vi "_PC_Daemon_Config_SaveData.vi"(8 "error in (no error)":errorcluster) -> (0 "error out":errorcluster)   [LabVIEW 2018]
uses:
  <vilib>/event_ctls.llb/eventvkey.ctl
panel:
  in  "Apply":bool
  in  "S/N":dbl
  in  "Noise Height":dbl
  in  "Auto Save":bool
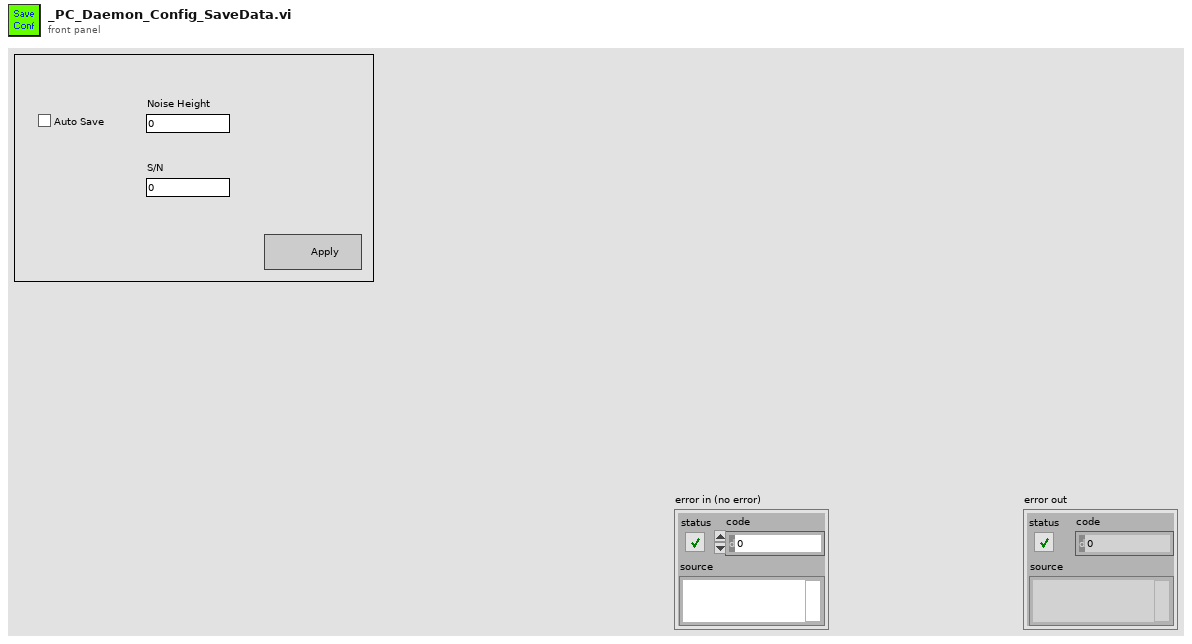
[diagram p1: front panel]
types:
  T1 = enum8{"Enabled", "Disabled", "Disabled and Grayed Out"}
  T2 = typedef "eventvkey.ctl" = enum16{"ASCII", "Enter", "Return", "Shift", "Ctrl", "Alt", "Cmd", "Opt", "Caps", "NumLock", "Clear", "Break", "Up", "Down", "Left", "Right", "Insert", "Delete", "Home", "End", "PageUp", "PageDown", "Escape", "Help", "Pause", "ScrollLock", "F1", "F2", "F3", "F4", "F5", "F6", "F7", "F8", "F9", "F10", "F11", "F12", "F13", "F14", "F15", "F16", "F17", "F18", "F19", "F20", "F21", "F22", "F23", "F24", "Play", "VolumeUp", "VolumeDown", "Mute", "Two Byte Char"}
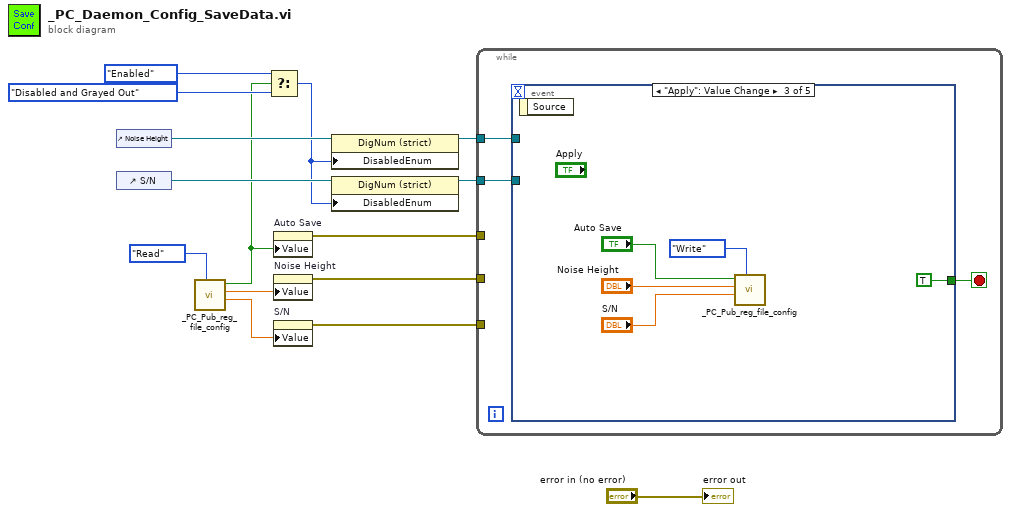
[diagram p0: block diagram]
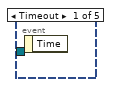
[diagram p2: hidden frame]
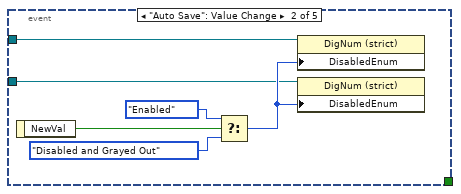
[diagram p3: hidden frame]
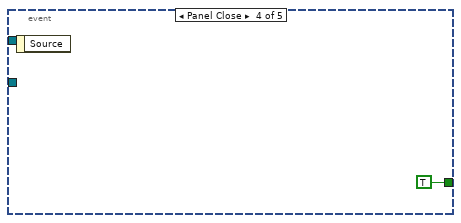
[diagram p4: hidden frame]
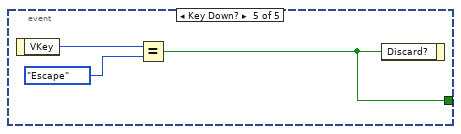
[diagram p5: hidden frame]
diagram:
  n1 = control-ref of="Noise Height"() -> (w8:refnum<vi>)
  n2 = control-ref of="S/N"() -> (w7:refnum<vi>)
  n3 = call "_PC_Pub_reg_file_config.vi"("func"=enum16{"None", "Write", "Read"}."Read") -> ("FileSN out"=w9:sgl, "FileNoise out"=w10:dbl, "AutoSave out"=w2:bool)  [unwired: 4 in, 1 out]
  n4 = Select(t=T1."Enabled" ("Disabled"), s=w2, f=T1."Disabled and Grayed Out" ("Disabled")) -> (s? t:f=w1:T1)
  n5 = property on="Auto Save" class="Bool (strict)"("Value"=w2) -> (error out=w15:errorcluster)  [unwired: 2 in, 1 out]
  n6 = property on="Noise Height" class="DigNum (strict)"("Value"=w10) -> (error out=w14:errorcluster)  [unwired: 2 in, 1 out]
  n7 = property on="S/N" class="DigNum (strict)"("Value"=w9) -> (error out=w13:errorcluster)  [unwired: 2 in, 1 out]
  n8 = property class="DigNum (strict)"(reference=w8, "DisabledEnum"=w1) -> (reference out=w5:refnum<vi>)  [unwired: 1 in, 1 out]
  n9 = property class="DigNum (strict)"(reference=w7, "DisabledEnum"=w1) -> (reference out=w6:refnum<vi>)  [unwired: 1 in, 1 out]
  n10 = while {
    tunnel: w15 -> [_]
    tunnel: w14 -> [_]
    tunnel: w13 -> [_]
    tunnel: w6 -> [w17]
    tunnel: w5 -> [w16]
    stop <- w18 stop-if-true
    n11 = event shown="[2] \"Apply\": Value Change" {
      selector: _ -> [_ _ _ _ _]
      dyn-events: _ -> [_ _ _ _ _]
      timeout: _ -> [_ _ _ _ _]
      tunnel: [_ _ TRUE TRUE w31] -> w18
      tunnel: w17 -> [_ w20 _ _ _]
      tunnel: w16 -> [_ w19 _ _ _]
      event Timeout {
        n12 = event-data() -> ()  [unwired: 1 in, 1 out]
      }
      event "Auto Save": Value Change {
        n13 = event-data() -> ("NewVal"=w24:bool)  [unwired: 1 in]
        n14 = Select(t=T1."Enabled" ("Disabled"), s=w24, f=T1."Disabled and Grayed Out" ("Disabled")) -> (s? t:f=w23:T1)
        n15 = property class="DigNum (strict)"(reference=w19, "DisabledEnum"=w23) -> ()  [unwired: 1 in, 2 out]
        n16 = property class="DigNum (strict)"(reference=w20, "DisabledEnum"=w23) -> ()  [unwired: 1 in, 2 out]
      }
      event "Apply": Value Change {
        n17 = event-data() -> ()  [unwired: 1 in, 1 out]
        n18 = call "_PC_Pub_reg_file_config.vi"("func"=enum16{"None", "Write", "Read"}."Write", "FileSN in"="S/N", "FileNoise in"="Noise Height", "AutoSave in"="Auto Save") -> ()  [unwired: 1 in, 4 out]
      }
      event Panel Close {
        n19 = event-data() -> ()  [unwired: 1 in, 1 out]
      }
      event Key Down? {
        n20 = event-data() -> ("VKey"=w33:T2)  [unwired: 1 in]
        n21 = Equal?(x=w33, y=eventvkey."Escape") -> (x = y?=w31:bool)
        n22 = event-data("Discard?"=w31) -> ()  [unwired: 1 in, 1 out]
      }
    }
  }
  "error out" <- "error in (no error)"
